vi "Request Data.vi"(6 "Qualifier":string, 8 "error in":errorcluster, 9 "notifier":refnum<notifier>, 10 "Data to Send":string, 11 "SwitchMatrix in":refnum<class "SwitchMatrix.lvclass">) -> (0 "error out":errorcluster, 3 "SwitchMatrix out":refnum<class "SwitchMatrix.lvclass">)   [LabVIEW 2019, in "SwitchMatrix.lvlib" / "SwitchMatrix.lvclass"]
doc: "Data to Send is a required input that describes the measurement or query function to be performed\nQualifier is a secondary variable used in the event that specificity must be provided to the query function\n****Note****\nIf further specificity is required, the qualifier must be used in a comma delimited format to increase the overall variable count. Additional specificity must be provided by the child class and interpreted by the automated call.\n\nnotifier is a single variant notifier in which the instrument will send the data notification to the automated tool."
uses:
  Library/SwitchMatrix.lvclass
  C:/Users/Public/Documents/Development/builds/Instruments/Instruments.lvlibp/Library/Instruments.lvclass
  builds/Instruments/Instruments.lvlibp/Private/Accessors/Read Poll(ms).vi
  builds/Instruments/Instruments.lvlibp/Private/Polymorphic/Special/Event from String.vi
  builds/Instruments/Instruments.lvlibp/Accessors/Command with Logging.vi
  builds/Instruments/Instruments.lvlibp/Library/Instruments.lvclass
  builds/Instruments/Instruments.lvlibp
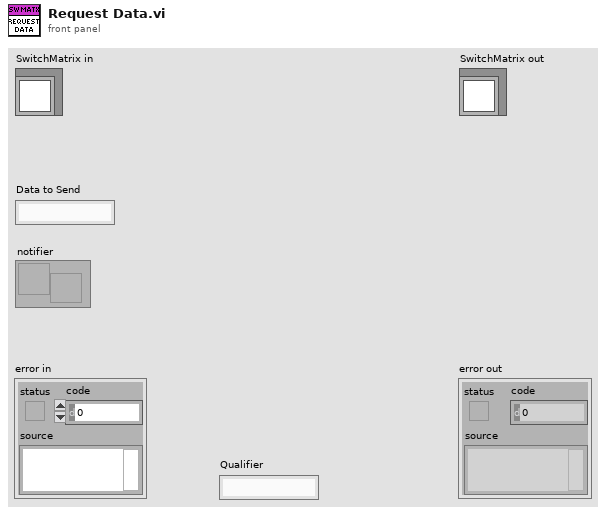
[diagram p1: front panel]
types:
  T1 = cluster{"Timestamp":timestamp, "Description":string, "Data":string}
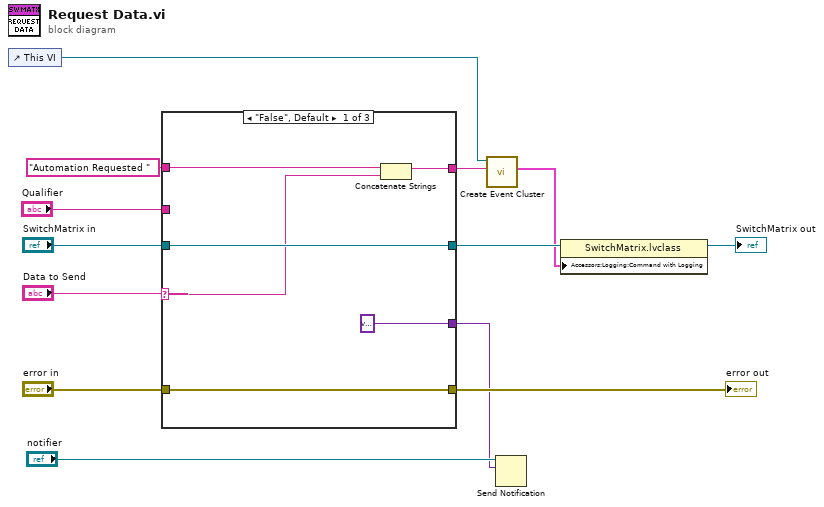
[diagram p0: block diagram]
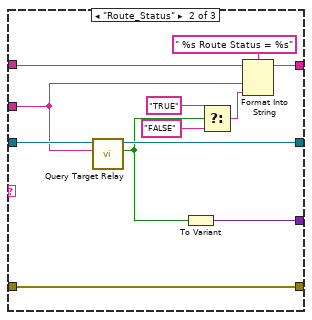
[diagram p2: hidden frame]
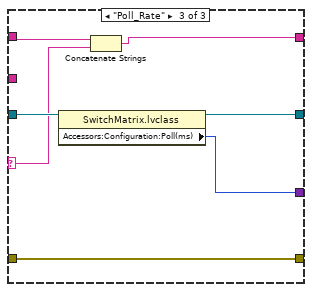
[diagram p3: hidden frame]
diagram:
  n1 = control-ref of="This VI"() -> (w5:refnum<vi>)
  n2 = case shown="\"False\", Default" "Data to Send" {
    selector: "Data to Send" -> [w14 _ w33]
    tunnel: "SwitchMatrix in" -> [w18 w29 w38]
    tunnel: "Qualifier" -> [_ w28 _]
    tunnel: "Automation Requested " -> [w15 w31 w34]
    tunnel: [w18 w27 w37] -> w4
    tunnel: [variant ("Variant") w25 w36] -> w6
    tunnel: [w19 w26 w35] -> w9
    tunnel: "error in" -> [w19 w26 w35]
    tunnel: [w16 w20 w32] -> w1
    frame "False", Default {
      n3 = Concatenate Strings(w15, w14) -> (w16:string)
    }
    frame "Route_Status" {
      n4 = call "Query Target Relay.vi"("Relay Name"=w28, "SwitchMatrix in"=w29) -> ("State"=w24:bool, "SwitchMatrix out"=w27:refnum<class "SwitchMatrix.lvclass">)  [unwired: 7 in, 1 out]
      n5 = To Variant(anything=w24) -> (Variant=w25:variant)
      n6 = Select(t="TRUE", s=w24, f="FALSE") -> (s? t:f=w21:string)
      n7 = Format Into String(format string=" %s Route Status = %s", initial string=w31, w28, w21) -> (resulting string=w20:string)  [unwired: 1 in, 1 out]
    }
    frame "Poll_Rate" {
      n8 = property class="SwitchMatrix.lvclass"(reference=w38) -> (reference out=w37:refnum<class "SwitchMatrix.lvclass">, "Accessors:Configuration:Poll(ms)"=w36:u32)  [unwired: 1 in, 1 out]
      n9 = Concatenate Strings(w34, w33) -> (w32:string)
    }
  }
  "error out" <- w9
  n10 = call-poly "Create Event Cluster.vi"("Value"=w1, "VI Refnum"=w5) -> ("Event Data"=w2:T1)  [unwired: 9 in]
  n11 = Send Notification(notification=w6, notifier="notifier") -> ()  [unwired: 1 in, 2 out]
  n12 = property class="SwitchMatrix.lvclass"(reference=w4, "Accessors:Logging:Command with Logging"=w2) -> (reference out=→"SwitchMatrix out":refnum<class "SwitchMatrix.lvclass">)  [unwired: 1 in, 1 out]
